vi "Test C.vi"(8 "error in (no error)":errorcluster) -> (0 "error out":errorcluster)   [LabVIEW 2019, in "Simple Example(Station1).lvlib"]
uses:
  Simple Example(Station1).lvlib
  b65cedc0-6f88-47fe-863c-f92be18f8f6a.vi
  941f3686-130e-45b0-8e30-bc4649ace6bb.vi
  Read Limit(String Array).vi
  LVUT Global 1.vi
  <vilib>/Utility/Data Type/Get Type Information.vi
  <vilib>/Utility/error.llb/Trim Whitespace.vi
  Equal Value.vi
  Unit Test Engine Tools.lvlib
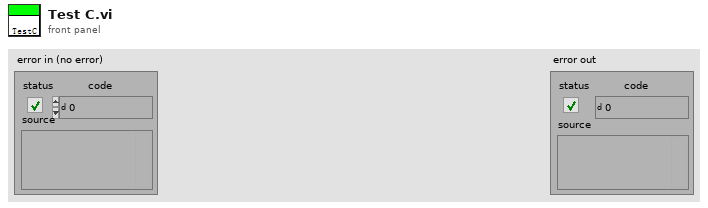
[diagram p1: front panel]
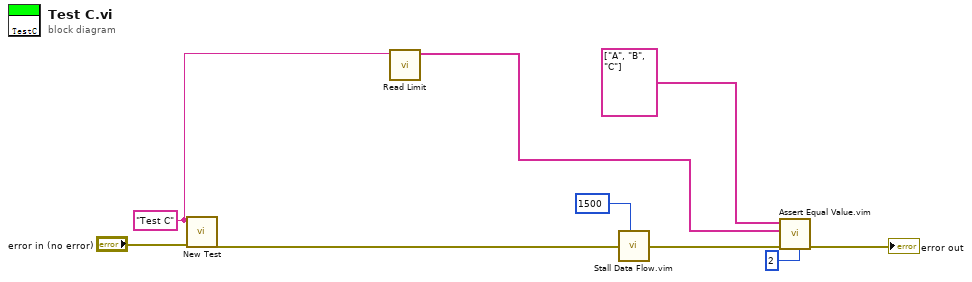
[diagram p0: block diagram]
diagram:
  w2 = "Test C" ("Test")
  n1 = call "New Test.vi"("error in (no error)"="error in (no error)", "Test"=w2) -> ("error out"=w8:errorcluster)  [unwired: 9 in]
  n2 = call-poly "Read Limit.vi"("Test"=w2) -> ("b"=w1:string[])  [unwired: 8 in, 2 out]
  n3 = call "Stall Data Flow.vim"("value in"=w8, "milliseconds to wait"=u32 1500) -> ("value out"=w5:errorcluster)  [unwired: 1 out]
  n4 = call "Assert Equal Value.vim"("precision (2)"=i16 2 ("precision (6)"), "error in (no error)"=w5, "Y"=w1, "X"=string[] ["A", "B", "C"]) -> ("error out"=→"error out":errorcluster)  [unwired: 7 in]
